vi "Execute.vi"(5 "SleepTerminalArray":refnum<vi>, 6 "ExeRef":refnum<vi>, 7 "ActiveTerminalArray":refnum<vi>, 8 "error in (no error)":errorcluster, 9 "Json_In":string, 10 "VariableRef":T2, 11 "Info":T1) -> (0 "Error Out":errorcluster, 1 "NumResultArray":dbl[](array[numeric]), 2 "StrResultArray":string[](array[string]), 3 "StrResult":string, 4 "NumResult":dbl)   [LabVIEW 2018, in "Dialog.lvlib"]
uses:
  Dialog.lvlib
  <userlib>/_OpenG.lib/dictionary/dictionary.llb/Dictionary Object RefNum__ogtk.ctl
  <userlib>/_OpenG.lib/dictionary/dictionary.llb/Dictionary Object RefNum - Enum__ogtk.ctl
  <vilib>/addons/_JKI.lib/Serialization/JSON/JKI JSON Serialization.lvlib
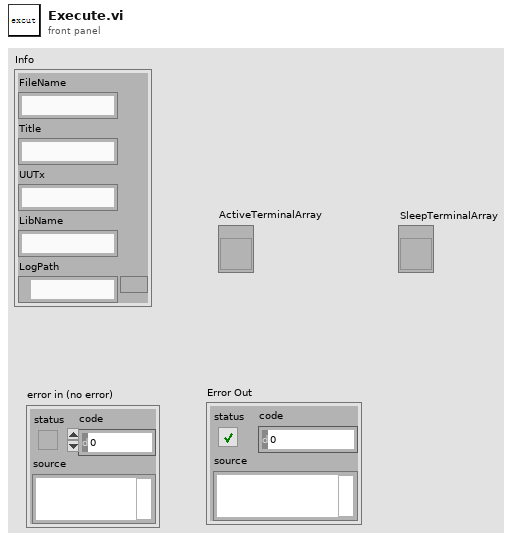
[diagram p1: front panel]
types:
  T1 = cluster{"FileName":string, "Title":string, "UUTx":string, "LibName":string, "LogPath":path}
  T2 = typedef "Dictionary Object RefNum__ogtk.ctl" = refnum<k1>
  T3 = cluster{"AlertDialog":cluster{"json":cluster{"Method":string, "Message":string, "PicName":string}}, "ConfirmDialog":cluster{"json":cluster{"Method":string, "Message":string, "PicName":string}}}
  T4 = cluster{"json":cluster{"Method":string, "Message":string, "PicName":string}}
  T5 = enum32{"invalid app kind", "Development System", "Run Time System", "Student Edition", "Embedded LabVIEW", "Evaluation", "Custom"}
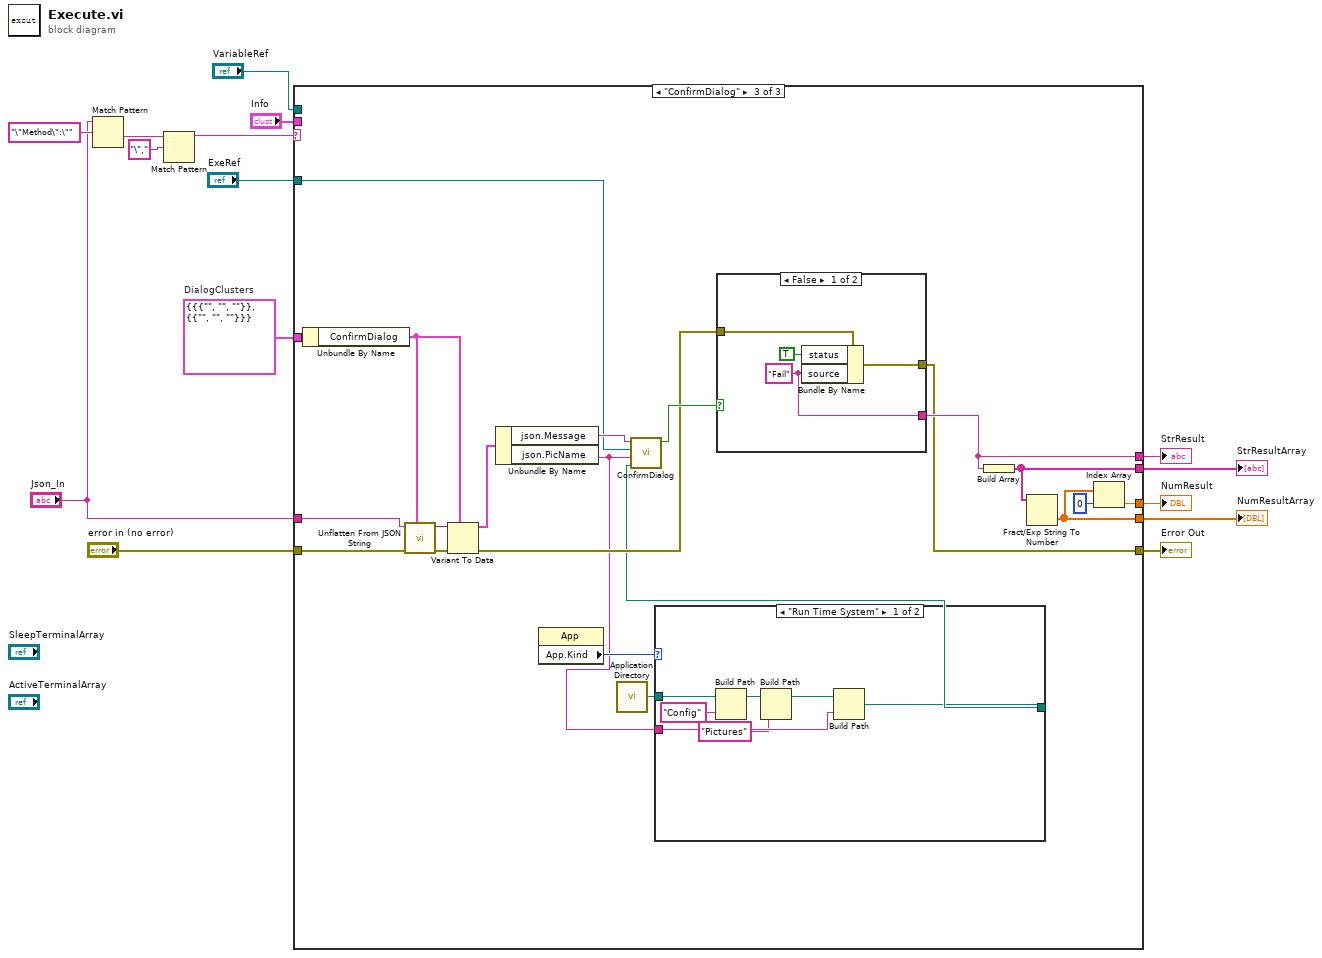
[diagram p0: block diagram]
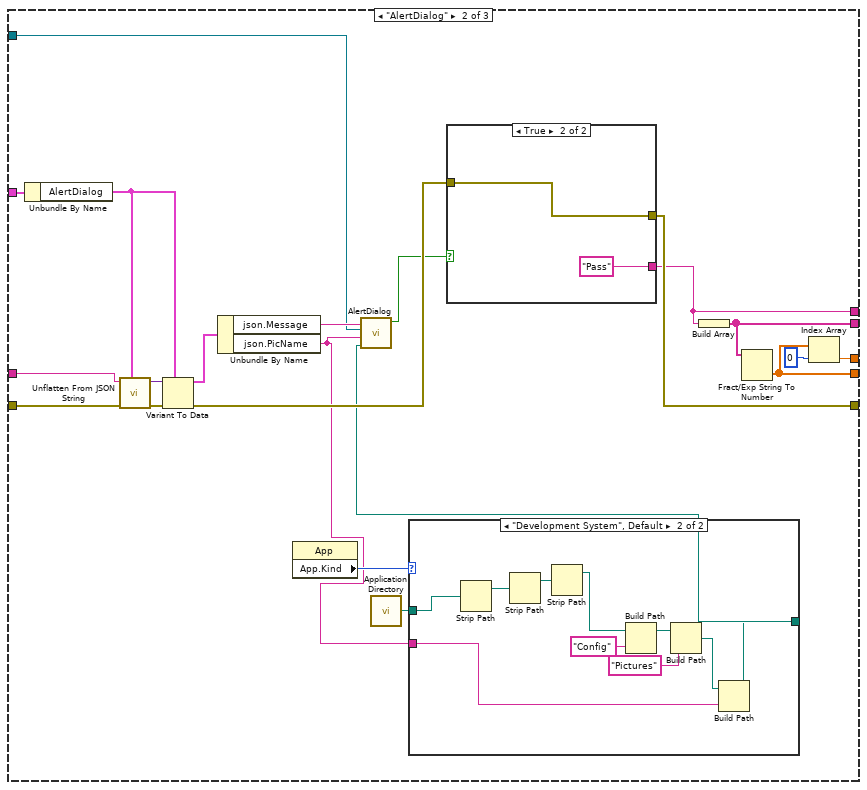
[diagram p3: hidden frame]
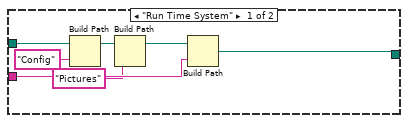
[diagram p4: hidden frame]
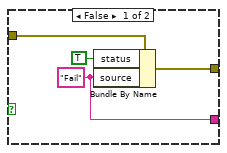
[diagram p5: hidden frame]
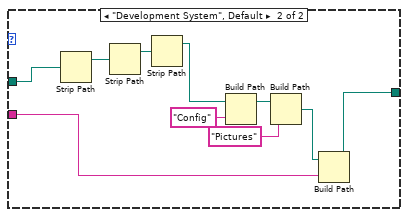
[diagram p6: hidden frame]
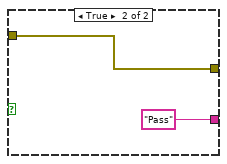
[diagram p7: hidden frame]
diagram:
  w2 = T3 {"AlertDialog"={"json"={"Method"="", "Message"="", "PicName"=""}}, "ConfirmDialog"={"json"={"Method"="", "Message"="", "PicName"=""}}}  # DialogClusters
  n1 = Match Pattern(string="Json_In", regular expression="\"Method\":\"") -> (after substring=w5:string)  [unwired: 1 in, 3 out]
  n2 = Match Pattern(string=w5, regular expression="\",") -> (before substring=w3:string)  [unwired: 1 in, 3 out]
  n3 = case shown="\"ConfirmDialog\"" w3 {
    tunnel: "Json_In" -> [_ w34 w78]
    tunnel: [w16 w22 w65] -> w15
    tunnel: "error in (no error)" -> [w16 w33 w77]
    tunnel: [_ w21 w66] -> w13
    tunnel: "VariableRef" -> [_ _ _]
    tunnel: [_ w27 w71] -> w12
    tunnel: [_ w30 w74] -> w11
    tunnel: [_ w32 w76] -> w10
    tunnel: "Info" -> [_ _ _]
    tunnel: w2 -> [_ w29 w73]
    tunnel: "ExeRef" -> [_ w25 w69]
    frame Default {
    }
    frame "AlertDialog" {
      n4 = Unbundle By Name(w29) -> ("AlertDialog"=w28:T4)
      n5 = call <vilib>:"Unflatten From JSON String.vi"("Type and Defaults"=w28, "error in (no error)"=w33, "JSON String"=w34) -> ("error out"=w36:errorcluster, "Variant"=w37:variant)  [unwired: 7 in]
      n6 = Variant To Data(error in=w36, type=w28, Variant=w37) -> (data=w35:T4, error out=w24:errorcluster)
      n7 = Unbundle By Name(w35) -> ("json.Message"=w26:string, "json.PicName"=w18:string)
      n8 = property class="App"() -> ("App.Kind"=w19:T5)  [unwired: 2 in, 2 out]
      n9 = call <vilib>:"Application Directory.vi"() -> ("Application Directory"=w20:path)
      n10 = case shown="\"Development System\", Default" w19 {
        tunnel: [w38 w52] -> w17
        tunnel: w20 -> [w44 w51]
        tunnel: w18 -> [w43 w50]
        frame "Run Time System" {
          n11 = Build Path(base path=w44, name or relative path="Config") -> (appended path=w42:path)
          n12 = Build Path(base path=w42, name or relative path="Pictures") -> (appended path=w40:path)
          n13 = Build Path(base path=w40, name or relative path=w43) -> (appended path=w38:path)
        }
        frame "Development System", Default {
          n14 = Strip Path(path=w51) -> (stripped path=w54:path)  [unwired: 1 out]
          n15 = Strip Path(path=w54) -> (stripped path=w53:path)  [unwired: 1 out]
          n16 = Strip Path(path=w53) -> (stripped path=w47:path)  [unwired: 1 out]
          n17 = Build Path(base path=w47, name or relative path="Config") -> (appended path=w49:path)
          n18 = Build Path(base path=w49, name or relative path="Pictures") -> (appended path=w45:path)
          n19 = Build Path(base path=w45, name or relative path=w50) -> (appended path=w52:path)
        }
      }
      n20 = call "AlertDialog.vi"("Path"=w17, "PicName"=w18, "VI Refnum"=w25, "提示"=w26) -> ("Result"=w23:bool)  [unwired: 7 in]
      n21 = case shown="True" w23 {
        tunnel: w24 -> [w58 w60]
        tunnel: [w56 w60] -> w22
        tunnel: [w55 "Pass"] -> w21
        frame False {
          w55 = "Fail" ("source")
          n22 = Bundle By Name(cluster=w58, "status"=TRUE, "source"=w55) -> (w56:errorcluster)
        }
        frame True {
        }
      }
      n23 = Build Array(w21) -> (w27:string[])
      n24 = Fract/Exp String To Number(string=w27) -> (number=w32:dbl[])  [unwired: 3 in, 1 out]
      n25 = Index Array(array=w32, index=0) -> (element=w30:dbl)
    }
    frame "ConfirmDialog" {
      n26 = Unbundle By Name(w73) -> ("ConfirmDialog"=w72:T4)
      n27 = call <vilib>:"Unflatten From JSON String.vi"("Type and Defaults"=w72, "error in (no error)"=w77, "JSON String"=w78) -> ("error out"=w80:errorcluster, "Variant"=w81:variant)  [unwired: 7 in]
      n28 = Variant To Data(error in=w80, type=w72, Variant=w81) -> (data=w79:T4, error out=w67:errorcluster)
      n29 = Unbundle By Name(w79) -> ("json.Message"=w70:string, "json.PicName"=w62:string)
      n30 = property class="App"() -> ("App.Kind"=w63:T5)  [unwired: 2 in, 2 out]
      n31 = call <vilib>:"Application Directory.vi"() -> ("Application Directory"=w64:path)
      n32 = case shown="\"Run Time System\"" w63 {
        tunnel: [w82 w96] -> w61
        tunnel: w64 -> [w88 w95]
        tunnel: w62 -> [w87 w94]
        frame "Run Time System" {
          n33 = Build Path(base path=w88, name or relative path="Config") -> (appended path=w86:path)
          n34 = Build Path(base path=w86, name or relative path="Pictures") -> (appended path=w84:path)
          n35 = Build Path(base path=w84, name or relative path=w87) -> (appended path=w82:path)
        }
        frame "Development System", Default {
          n36 = Strip Path(path=w95) -> (stripped path=w98:path)  [unwired: 1 out]
          n37 = Strip Path(path=w98) -> (stripped path=w97:path)  [unwired: 1 out]
          n38 = Strip Path(path=w97) -> (stripped path=w91:path)  [unwired: 1 out]
          n39 = Build Path(base path=w91, name or relative path="Config") -> (appended path=w93:path)
          n40 = Build Path(base path=w93, name or relative path="Pictures") -> (appended path=w89:path)
          n41 = Build Path(base path=w89, name or relative path=w94) -> (appended path=w96:path)
        }
      }
      n42 = call "ConfirmDialog.vi"("Path"=w61, "PicName"=w62, "VI Refnum"=w69, "提示"=w70) -> ("Result"=w68:bool)  [unwired: 7 in]
      n43 = case shown="False" w68 {
        tunnel: w67 -> [w102 w104]
        tunnel: [w100 w104] -> w65
        tunnel: [w99 "Pass"] -> w66
        frame False {
          w99 = "Fail" ("source")
          n44 = Bundle By Name(cluster=w102, "status"=TRUE, "source"=w99) -> (w100:errorcluster)
        }
        frame True {
        }
      }
      n45 = Build Array(w66) -> (w71:string[])
      n46 = Fract/Exp String To Number(string=w71) -> (number=w76:dbl[])  [unwired: 3 in, 1 out]
      n47 = Index Array(array=w76, index=0) -> (element=w74:dbl)
    }
  }
  "StrResult" <- w13
  "Error Out" <- w15
  "StrResultArray" <- w12
  "NumResult" <- w11
  "NumResultArray" <- w10
